vi "BITCOUNT.vi"(0 "refnum in":refnum<vi>, 1 "Key":string, 5 "Use [Start - End] ?":bool, 7 "Start":string, 11 "error in":errorcluster, 13 "End":string) -> (4 "refnum out":refnum<vi>, 6 "Data":T1, 15 "error out":errorcluster)   [LabVIEW 2023]
uses:
  SubVIs/Controls/redis-data.ctl
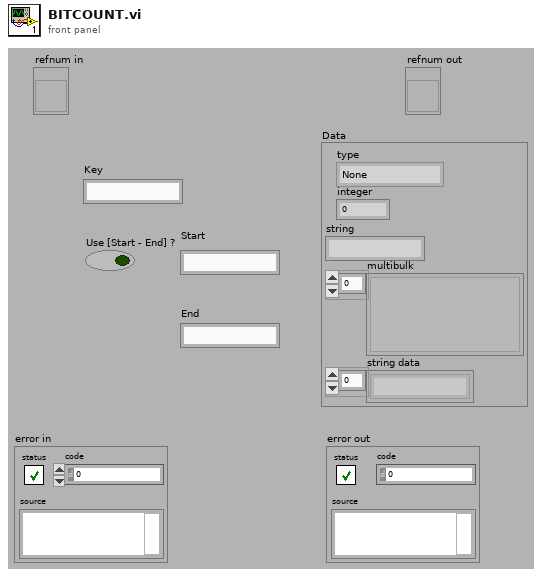
[diagram p1: front panel]
types:
  T1 = typedef "redis-data.ctl" = cluster{"type":enum16{"None", "Error", "Status", "Nil", "Integer", "String", "Multibulk"}, "integer":i64, "string":string, "multibulk":variant[], "string data":string[]}
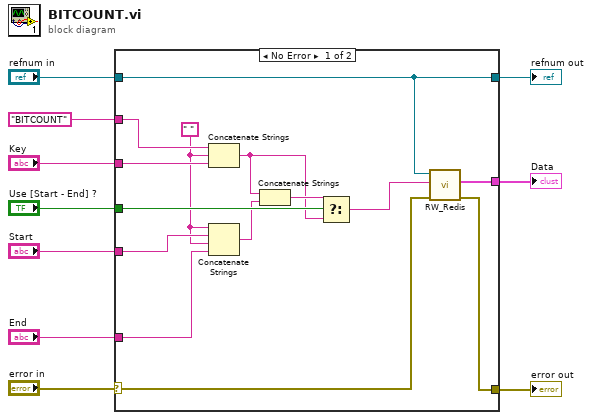
[diagram p0: block diagram]
diagram:
  n1 = case shown="No Error" "error in" {
    selector: "error in" -> [w23 w26]
    tunnel: "Key" -> [w20 _]
    tunnel: "BITCOUNT" -> [w24 _]
    tunnel: "refnum in" -> [w14 w25]
    tunnel: [w22 w26] -> w8
    tunnel: [w21 _] -> w1
    tunnel: "Start" -> [w19 _]
    tunnel: "Use [Start - End] ?" -> [w18 _]
    tunnel: "End" -> [w12 _]
    tunnel: [w14 w25] -> w3
    frame No Error {
      w13 = " "
      n2 = Concatenate Strings(w24, w13, w20) -> (w16:string)
      n3 = Concatenate Strings(w13, w19, w13, w12) -> (w15:string)
      n4 = Concatenate Strings(w16, w15) -> (w17:string)
      n5 = Select(t=w17, s=w18, f=w16) -> (s? t:f=w11:string)
      n6 = call "RW_Redis.vi"("error in"=w23, "command"=w11, "TCP session in"=w14) -> ("error out"=w22:errorcluster, "Data"=w21:T1)  [unwired: 6 in, 1 out]
    }
    frame Error {
    }
  }
  "error out" <- w8
  "Data" <- w1
  "refnum out" <- w3
